vi "Read Bus Controller.vi"(6 "parameters file version":string, 8 "error in":errorcluster, 11 "channel ref in":refnum<k20>) -> (0 "error out":errorcluster, 1 "bus controller name":string, 2 "add bus controller":bool=TRUE, 3 "channel ref out":refnum<k20>)   [LabVIEW 2020, in "MIL-STD 1553 Import.lvlib"]
uses:
  MIL-STD 1553 Import.lvlib
  829340a0-7361-4f55-8ea4-c564bd074793.vi
  c51f0b55-bb46-4a24-bf1d-89c645bb4080.vi
  3e5c2c5e-523c-4bba-a9cb-8720dcec4f9c.vi
  a7defcbe-187e-4554-abff-804d775517eb.vi
  829340a0-7361-4f55-8ea4-c564bd074793.vi/b1e6fcf8-dac1-42d2-b1fe-151afe06dbd4.vi
  c51f0b55-bb46-4a24-bf1d-89c645bb4080.vi/b1e6fcf8-dac1-42d2-b1fe-151afe06dbd4.vi
  3e5c2c5e-523c-4bba-a9cb-8720dcec4f9c.vi/b1e6fcf8-dac1-42d2-b1fe-151afe06dbd4.vi
  a7defcbe-187e-4554-abff-804d775517eb.vi/b1e6fcf8-dac1-42d2-b1fe-151afe06dbd4.vi
  3e5c2c5e-523c-4bba-a9cb-8720dcec4f9c.vi/b1e6fcf8-dac1-42d2-b1fe-151afe06dbd4.vi/49c1b1ee-2d2a-4a85-8ca5-42123c34e85a.vi
  Constants.vi
  <vilib>/xml/Get Node Text Content.vi
  <vilib>/Utility/error.llb/Error Cluster From Error Code.vi
  Scripting/Constants.vi
  Scripting/Ballard MIL-STD-1553 Scripting.lvlib
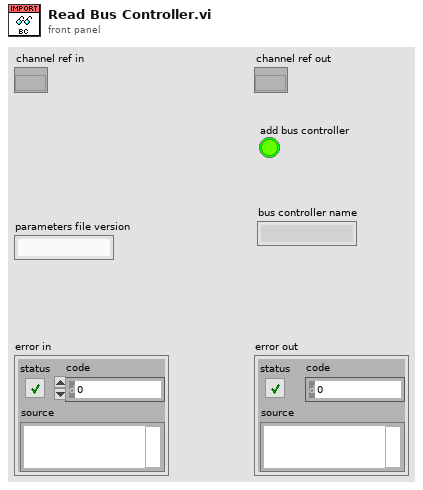
[diagram p1: front panel]
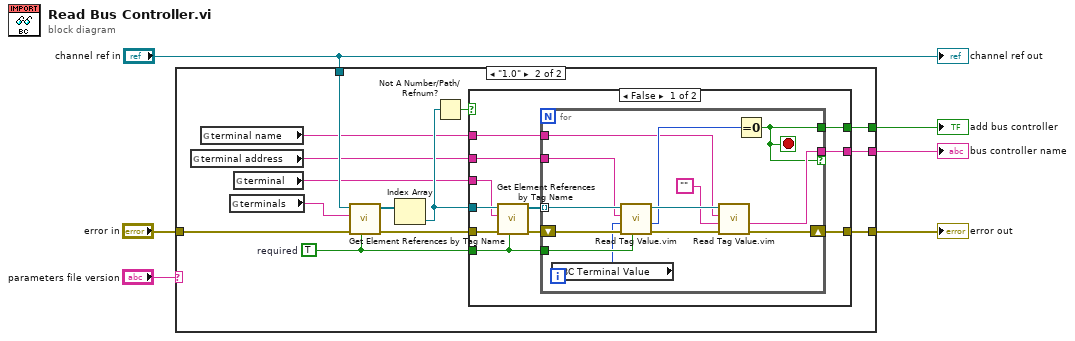
[diagram p0: block diagram]
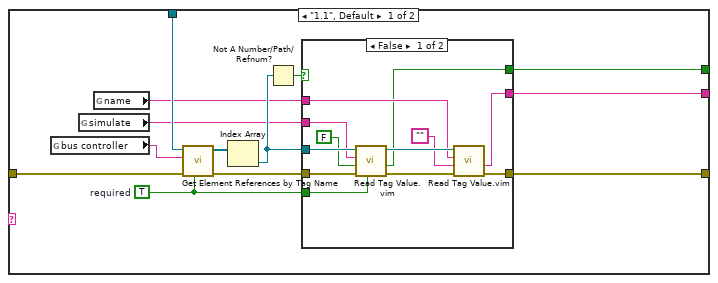
[diagram p2: hidden frame]
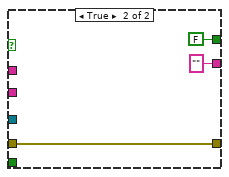
[diagram p3: hidden frame]
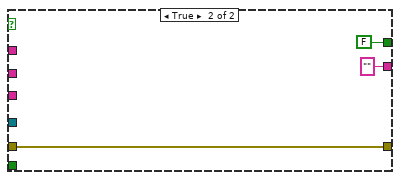
[diagram p4: hidden frame]
diagram:
  n1 = case shown="\"1.0\"" "parameters file version" {
    tunnel: [w19 w48] -> w6
    tunnel: "channel ref in" -> [w18 w47]
    tunnel: [w9 w38] -> w4
    tunnel: "error in" -> [w8 w37]
    tunnel: [w7 w36] -> w1
    frame "1.1", Default {
      w13 = TRUE  # required
      n2 = global read "Constants.vi" "bus controller"() -> (w12:string)
      n3 = global read "Constants.vi" "simulate"() -> (w11:string)
      n4 = global read "Constants.vi" "name"() -> (w10:string)
      n5 = call "Get Element References by Tag Name.vi"("required (F)"=w13, "error in"=w8, "tag name"=w12, "node in"=w18) -> ("error out"=w16:errorcluster, "array of elements"=w17:refnum<k20>[])  [unwired: 6 in]
      n6 = Index Array(array=w17) -> (element=w14:refnum<k20>)  [unwired: 1 in]
      n7 = Not A Number/Path/Refnum?(number/path/refnum=w14) -> (NaN/Path/Refnum?=w15:bool)
      n8 = case shown="False" w15 {
        tunnel: [w22 w34] -> w19
        tunnel: w14 -> [w30 _]
        tunnel: w16 -> [w31 w34]
        tunnel: w13 -> [w27 _]
        tunnel: w11 -> [w29 _]
        tunnel: w10 -> [w23 _]
        tunnel: [w21 FALSE ("value")] -> w9
        tunnel: [w20 "" ("value")] -> w7
        frame False {
          n9 = call "Read Tag Value.vim"("required (F)"=w27, "error in"=w31, "default"=FALSE, "tag name"=w29, "node in"=w30) -> ("error out"=w26:errorcluster, "value"=w21:bool, "node out"=w25:refnum<k20>)  [unwired: 4 in]
          n10 = call "Read Tag Value.vim"("error in"=w26, "default"="", "tag name"=w23, "node in"=w25) -> ("error out"=w22:errorcluster, "value"=w20:string)  [unwired: 5 in, 1 out]
        }
        frame True {
        }
      }
    }
    frame "1.0" {
      w42 = TRUE  # required
      n11 = global read "Constants.vi" "terminal address"() -> (w39:string)
      n12 = global read "Constants.vi" "terminal name"() -> (w35:string)
      n13 = global read "Constants.vi" "terminals"() -> (w41:string)
      n14 = global read "Constants.vi" "terminal"() -> (w40:string)
      n15 = call "Get Element References by Tag Name.vi"("required (F)"=w42, "error in"=w37, "tag name"=w41, "node in"=w47) -> ("error out"=w45:errorcluster, "array of elements"=w46:refnum<k20>[])  [unwired: 6 in]
      n16 = Index Array(array=w46) -> (element=w43:refnum<k20>)  [unwired: 1 in]
      n17 = Not A Number/Path/Refnum?(number/path/refnum=w43) -> (NaN/Path/Refnum?=w44:bool)
      n18 = case shown="False" w44 {
        tunnel: [w53 w75] -> w48
        tunnel: w43 -> [w58 _]
        tunnel: w45 -> [w57 w75]
        tunnel: w42 -> [w52 _]
        tunnel: w40 -> [w56 _]
        tunnel: w39 -> [w59 _]
        tunnel: [w51 FALSE ("value")] -> w38
        tunnel: [w50 "" ("value")] -> w36
        tunnel: w35 -> [w49 _]
        frame False {
          n19 = call "Get Element References by Tag Name.vi"("required (F)"=w52, "error in"=w57, "tag name"=w56, "node in"=w58) -> ("error out"=w54:errorcluster, "array of elements"=w55:refnum<k20>[])  [unwired: 6 in]
          n20 = for {
            tunnel: w59 -> [w67]
            tunnel: w55 -> [w68] mode=indexing
            shift-right: [w62] -> w53
            shift-left: w54 -> [w69]
            tunnel: w52 -> [w66]
            tunnel: [w63] -> w51
            tunnel: [w64] -> w50 if=w63
            tunnel: w49 -> [w61]
            stop <- w63 stop-if-true
            n21 = global read "Constants.vi" "BC Terminal Value"() -> (w60:u16)
            n22 = call "Read Tag Value.vim"("required (F)"=w66, "error in"=w69, "default"=w60, "tag name"=w67, "node in"=w68) -> ("error out"=w72:errorcluster, "value"=w65:u16, "node out"=w71:refnum<k20>)  [unwired: 4 in]
            n23 = call "Read Tag Value.vim"("error in"=w72, "default"="", "tag name"=w61, "node in"=w71) -> ("error out"=w62:errorcluster, "value"=w64:string)  [unwired: 5 in, 1 out]
            n24 = Equal To 0?(x=w65) -> (x = 0?=w63:bool)
          }
        }
        frame True {
        }
      }
    }
  }
  "error out" <- w6
  "add bus controller" <- w4
  "bus controller name" <- w1
  "channel ref out" <- "channel ref in"
